vi "CRYReport Part TX LIB.vi"(6 "Control Ref":refnum<k7>, 7 "sAction":string, 8 "nData":i32, 9 "sData":string, 10 "TXTextControl":refnum<k7>, 11 "cFrame":T1) -> (0 "nData_Out":i32, 1 "sData_Out":string, 3 "cFrame_Out":T1)   [LabVIEW 2013]
uses:
  CRYReport Global.vi
  CRYWindow/SubVI/CRYMain Sub Window Global.vi
  PrintTxDocDLL.dll
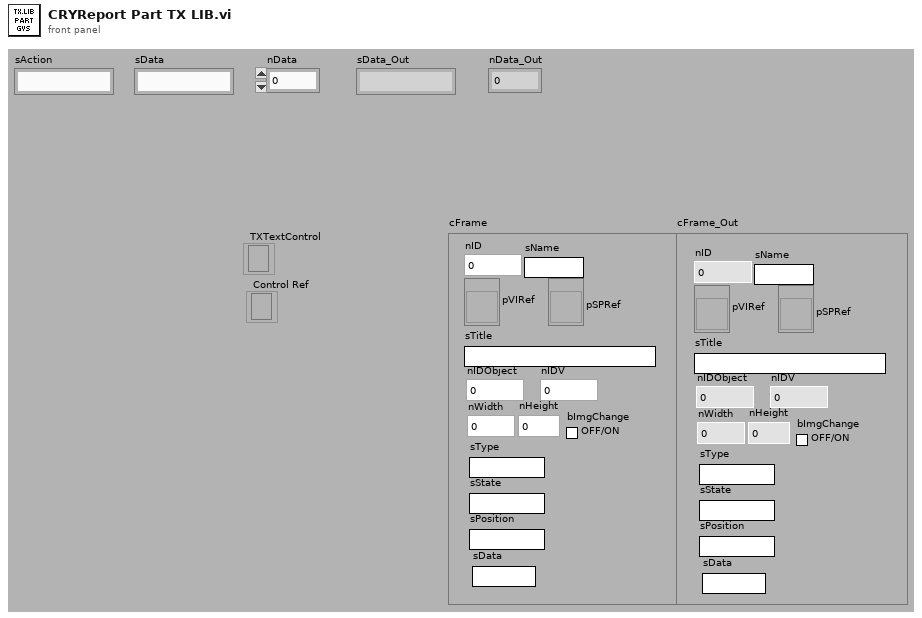
[diagram p1: front panel]
types:
  T1 = cluster{"nID":i16, "sName":string, "pVIRef":refnum<vi>, "pSPRef":refnum<vi>, "sTitle":string, "nIDObject":i16, "nIDV":i16, "nWidth":i16, "nHeight":i16, "bImgChange":bool, "sType":string, "sState":string, "sPosition":string, "sData":string}
  T2 = typedef "LVRectTypeDef.ctl" = cluster{"Left":i16, "Top":i16, "Right":i16, "Bottom":i16}
  T3 = cluster{"nType":i32, "nParent":i32, "pVIW":refnum<vi>, "pSPW":refnum<vi>, "nTypeF":i32, "pVIF":refnum<vi>, "pSPF":refnum<vi>, "nIDSpliter":i32, "nProperty":i32, "Bound":T2, "nID":i32, "nData":i32, "sData":string, "pWVI":refnum<vi>, "sTitle":string, "cPages":cluster{"nPage":i32, "sTitle":string, "sIcon":string, "pVI":refnum<vi>, "nID":i32}[], "pTab":refnum<vi>, "nIDPages":i32[], "pSPT":refnum<vi>, "sTemp":string, "nDockID":i32, "nDockLR":i32, "sIcon":string}
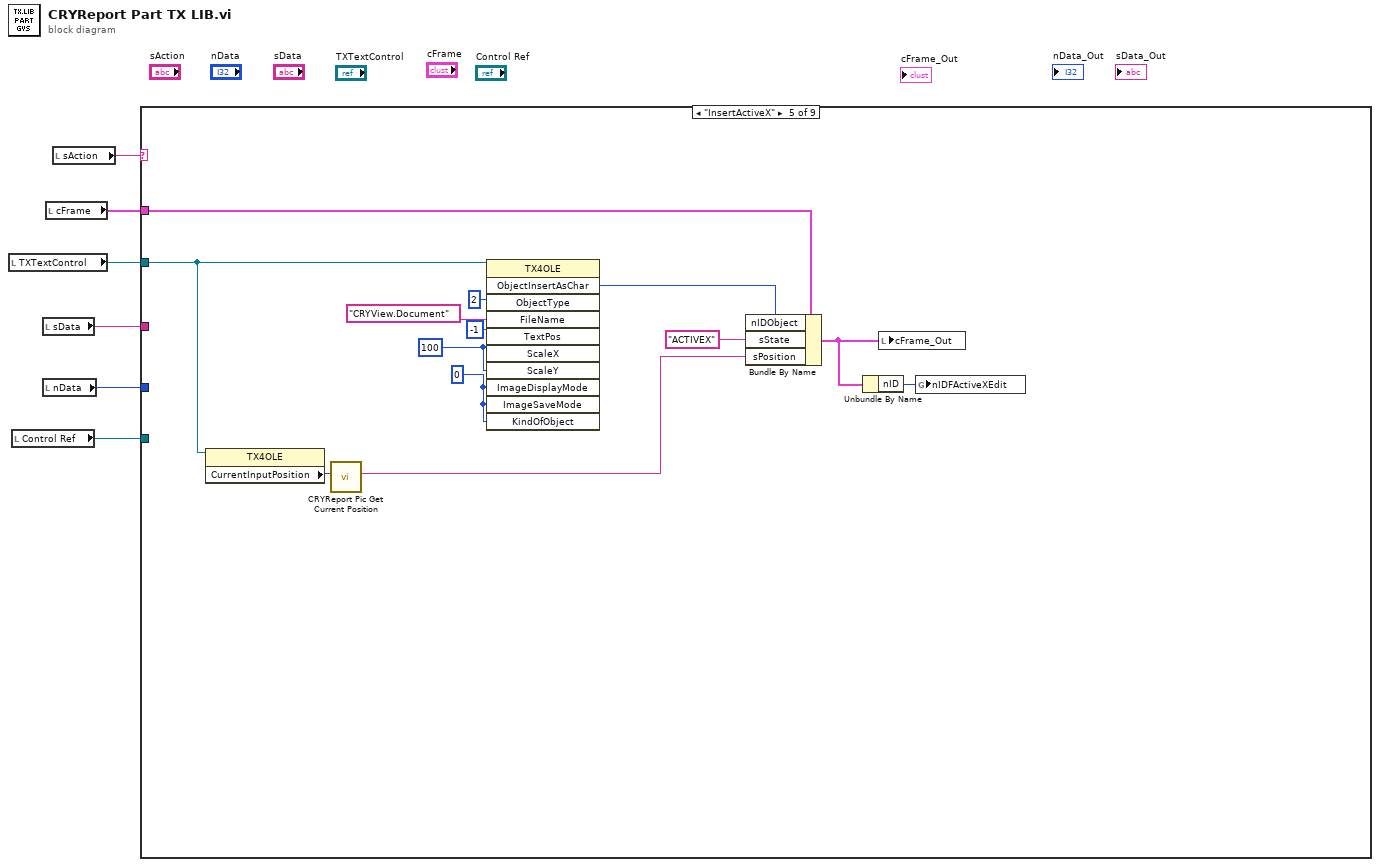
[diagram p0: block diagram]
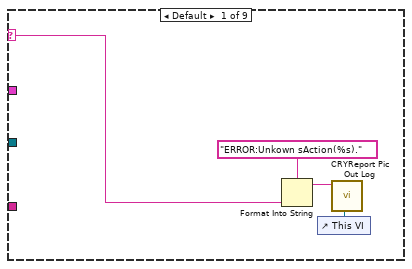
[diagram p2: hidden frame]
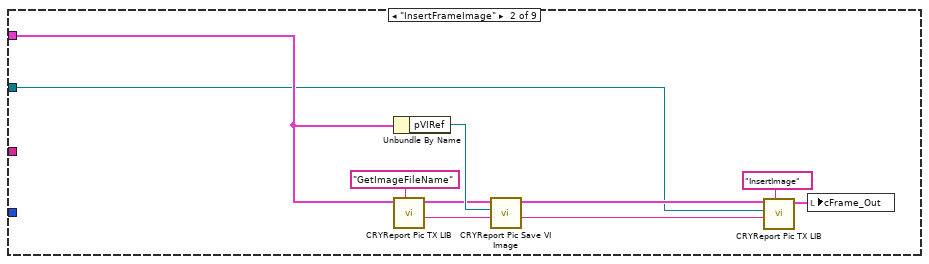
[diagram p3: hidden frame]
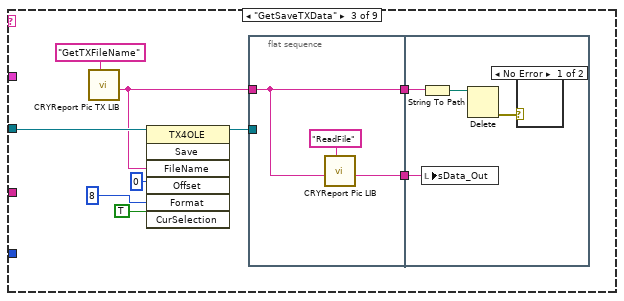
[diagram p4: hidden frame]
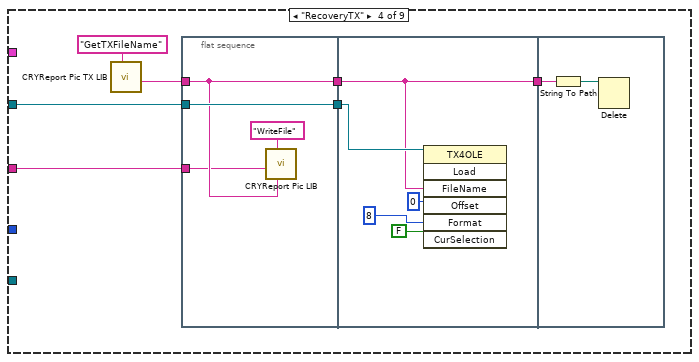
[diagram p6: hidden frame]
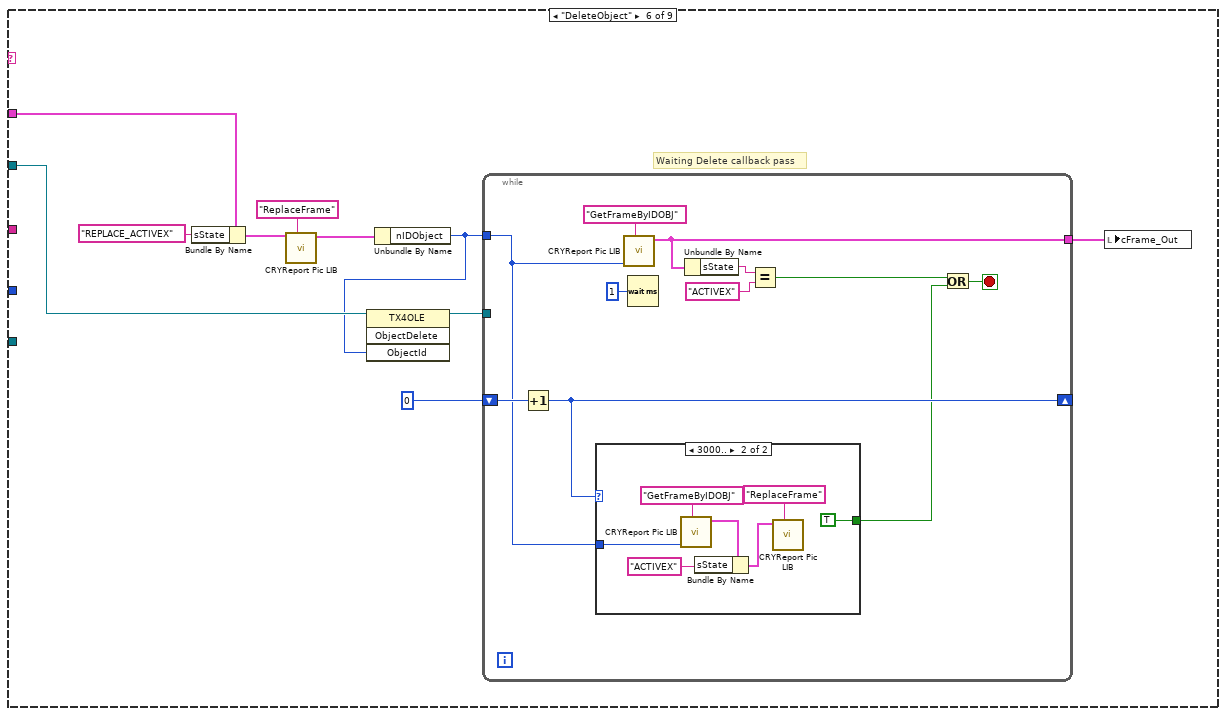
[diagram p7: hidden frame]
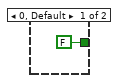
[diagram p8: hidden frame]
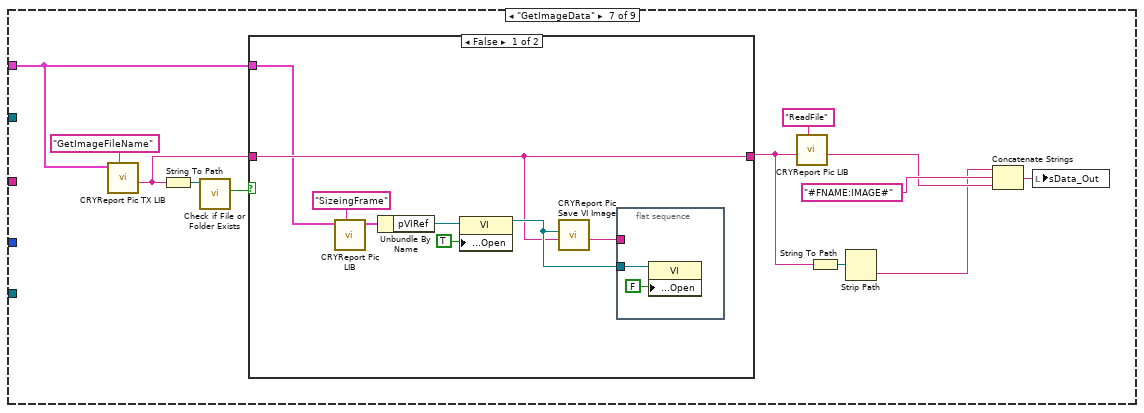
[diagram p9: hidden frame]
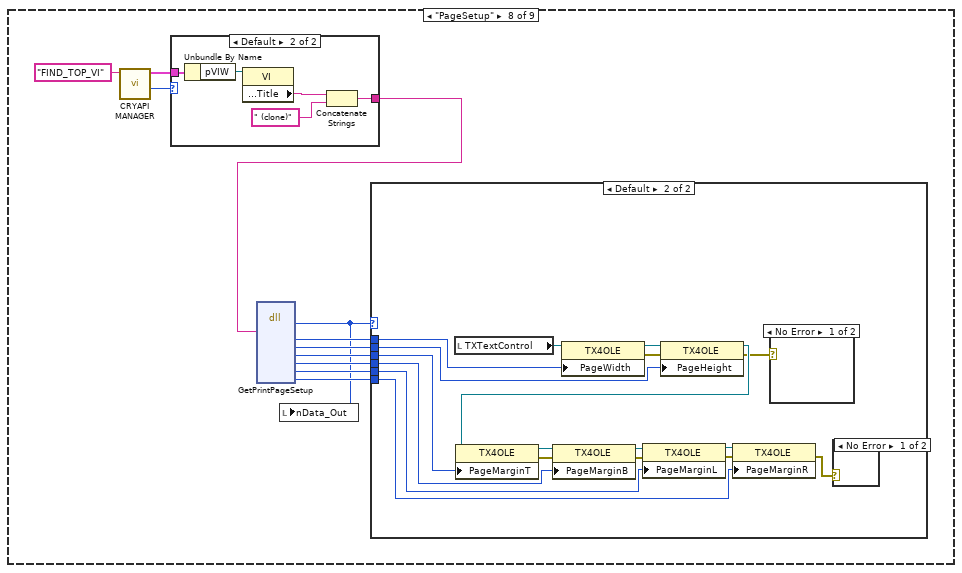
[diagram p11: hidden frame]
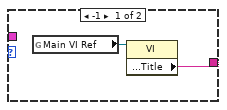
[diagram p15: hidden frame]
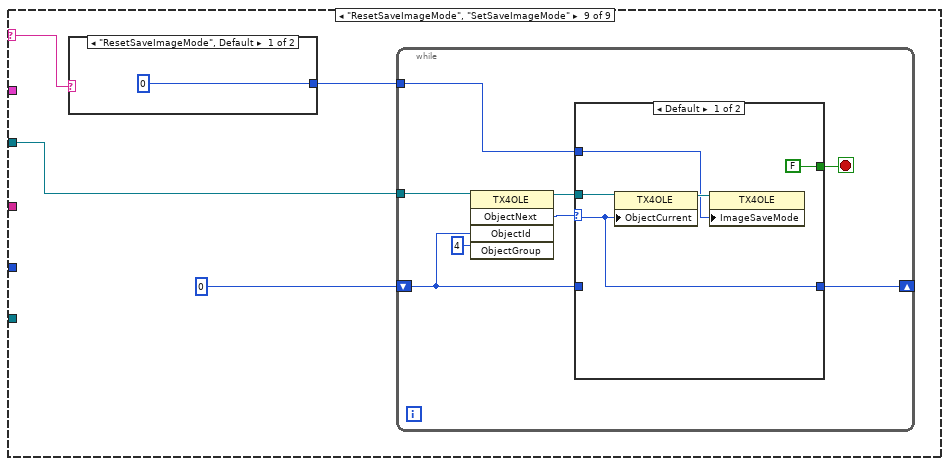
[diagram p16: hidden frame]
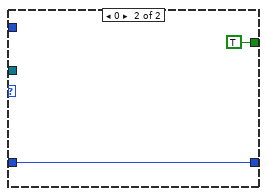
[diagram p17: hidden frame]
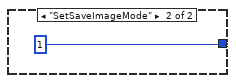
[diagram p18: hidden frame]
diagram:
  n1 = local read "TXTextControl"() -> (w2:refnum<k7>)
  n2 = local read "Control Ref"() -> (w1:refnum<k7>)
  n3 = local read "sData"() -> (w5:string)
  n4 = local read "nData"() -> (w4:i32)
  n5 = local read "cFrame"() -> (w3:T1)
  n6 = local read "sAction"() -> (w6:string)
  n7 = case shown="\"InsertActiveX\"" w6 {
    selector: w6 -> [w8 _ _ _ _ _ _ _ w159]
    tunnel: w5 -> [_ _ _ w41 _ _ _ _ _]
    tunnel: w4 -> [_ _ _ _ _ _ _ _ _]
    tunnel: w3 -> [_ w20 _ _ w56 w73 w105 _ _]
    tunnel: w2 -> [_ w15 w27 w40 w55 w74 _ _ w158]
    tunnel: w1 -> [_ _ _ _ _ _ _ _ _]
    frame Default {
      n8 = Format Into String(format string="ERROR:Unkown sAction(%s).", w8) -> (resulting string=w7:string)  [unwired: 2 in, 1 out]
      n9 = control-ref of="This VI"() -> (w10:refnum<vi>)
      n10 = call "CRYReport Pic Out Log.vi"("vi reference"=w10, "sData"=w7) -> ()  [unwired: 10 in]
    }
    frame "InsertFrameImage" {
      n11 = Unbundle By Name(w20) -> ("pVIRef"=w14:refnum<vi>)
      n12 = call "CRYReport Pic TX LIB.vi"("sAction"="GetImageFileName", "cFrame"=w20) -> ("sData_Out"=w12:string, "cFrame_Out"=w11:T1)  [unwired: 7 in, 1 out]
      n13 = call "CRYReport Pic Save VI Image.vi"("sData"=w12, "pVIRef"=w14, "cFrame"=w11) -> ("sData_Out"=w19:string, "cFrame_Out"=w18:T1)  [unwired: 7 in]
      n14 = call "CRYReport Pic TX LIB.vi"("sAction"="InsertImage", "sData"=w19, "TXTextControl"=w15, "cFrame"=w18) -> ("cFrame_Out"=w16:T1)  [unwired: 5 in, 2 out]
      n15 = local write "cFrame_Out"(w16) -> ()
    }
    frame "GetSaveTXData" {
      n16 = call "CRYReport Pic TX LIB.vi"("sAction"="GetTXFileName") -> ("sData_Out"=w24:string)  [unwired: 8 in, 2 out]
      n17 = invoke class="TX4OLE" method="Save"(reference=w27, "FileName"=w24, "Offset"=0, "Format"=8 ("nData"), "CurSelection"=TRUE) -> (reference out=w23:refnum<k7>)  [unwired: 2 in, 6 out]
      n18 = flat-sequence {
        tunnel: w24 -> [w31]
        tunnel: w23 -> [_]
        tunnel: [w31] -> w22
        tunnel: [w30] -> w21
        tunnel: w22 -> [w36]
        tunnel: w21 -> [w34]
        frame #0 {
          n19 = call "CRYReport Pic LIB.vi"("sAction"="ReadFile", "sData"=w31) -> ("sData_Out"=w30:string)  [unwired: 6 in, 3 out]
        }
        frame #1 {
          n20 = String To Path(string=w36) -> (path=w35:path)
          n21 = local write "sData_Out"(w34) -> ()
          n22 = Delete(path (use dialog)=w35) -> (error out=w33:errorcluster)  [unwired: 4 in, 2 out]
          n23 = case shown="No Error" w33 {
            frame No Error {
            }
            frame Error {
            }
          }
        }
      }
    }
    frame "RecoveryTX" {
      n24 = call "CRYReport Pic TX LIB.vi"("sAction"="GetTXFileName") -> ("sData_Out"=w42:string)  [unwired: 8 in, 2 out]
      n25 = flat-sequence {
        tunnel: w41 -> [w44]
        tunnel: w42 -> [w45]
        tunnel: w40 -> [w47]
        tunnel: [w45] -> w39
        tunnel: [w47] -> w38
        tunnel: w39 -> [w48]
        tunnel: w38 -> [w49]
        tunnel: [w48] -> w37
        tunnel: w37 -> [w53]
        frame #0 {
          n26 = call "CRYReport Pic LIB.vi"("sOption"=w45, "sAction"="WriteFile", "sData"=w44) -> ()  [unwired: 5 in, 4 out]
        }
        frame #1 {
          n27 = invoke class="TX4OLE" method="Load"(reference=w49, "FileName"=w48, "Offset"=0, "Format"=8 ("nData"), "CurSelection"=FALSE) -> ()  [unwired: 2 in, 7 out]
        }
        frame #2 {
          n28 = String To Path(string=w53) -> (path=w54:path)
          n29 = Delete(path (use dialog)=w54) -> ()  [unwired: 4 in, 3 out]
        }
      }
    }
    frame "InsertActiveX" {
      w62 = i16 0 ("ImageDisplayMode")
      w63 = i16 100 ("ScaleX")
      n30 = property class="TX4OLE"(reference=w55) -> ("CurrentInputPosition"=w57:variant)  [unwired: 1 in, 2 out]
      n31 = call "CRYReport Pic Get Current Position.vi"("CurrentInputPosition"=w57) -> ("sData_Out"=w61:string)  [unwired: 9 in, 1 out]
      n32 = invoke class="TX4OLE" method="ObjectInsertAsChar"(reference=w55, "ObjectType"=2, "FileName"="CRYView.Document", "TextPos"=-1, "ScaleX"=w63, "ScaleY"=w63, "ImageDisplayMode"=w62, "ImageSaveMode"=w62, "KindOfObject"=w62) -> ("ObjectInsertAsChar"=w67:i16)  [unwired: 2 in, 10 out]
      n33 = Bundle By Name(cluster=w56, "nIDObject"=w67, "sState"="ACTIVEX", "sPosition"=w61) -> (w59:T1)
      n34 = Unbundle By Name(w59) -> ("nID"=w58:i16)
      n35 = local write "cFrame_Out"(w59) -> ()
      n36 = global write "CRYReport Global.vi" "nIDFActiveXEdit"(w58) -> ()
    }
    frame "DeleteObject" {
      # "Waiting Delete callback pass"
      n37 = Bundle By Name(cluster=w73, "sState"="REPLACE_ACTIVEX") -> (w76:T1)
      n38 = call "CRYReport Pic LIB.vi"("sAction"="ReplaceFrame", "cFrame"=w76) -> ("cFrame_Out"=w72:T1)  [unwired: 6 in, 3 out]
      n39 = Unbundle By Name(w72) -> ("nIDObject"=w70:i16)
      n40 = invoke class="TX4OLE" method="ObjectDelete"(reference=w74, "ObjectId"=w70) -> (reference out=w71:refnum<k7>)  [unwired: 2 in, 3 out]
      n41 = while {
        tunnel: w71 -> [_]
        tunnel: w70 -> [w81]
        tunnel: [w84] -> w69
        shift-right: [w82] -> _
        shift-left: 0 -> [w83]
        stop <- w80 stop-if-true
        n42 = Increment(x=w83) -> (x+1=w82:i32)
        n43 = case shown="3000.." w82 {
          tunnel: w81 -> [_ w95]
          tunnel: [FALSE TRUE] -> w78
          frame 0, Default {
          }
          frame 3000.. {
            n44 = call "CRYReport Pic LIB.vi"("sAction"="GetFrameByIDOBJ", "nData"=w95) -> ("cFrame_Out"=w94:T1)  [unwired: 6 in, 3 out]
            n45 = Bundle By Name(cluster=w94, "sState"="ACTIVEX") -> (w91:T1)
            n46 = call "CRYReport Pic LIB.vi"("sAction"="ReplaceFrame", "cFrame"=w91) -> ()  [unwired: 6 in, 4 out]
          }
        }
        n47 = call "CRYReport Pic LIB.vi"("sAction"="GetFrameByIDOBJ", "nData"=w81) -> ("cFrame_Out"=w84:T1)  [unwired: 6 in, 3 out]
        n48 = Wait (ms)(milliseconds to wait=u32 1) -> ()  [unwired: 1 out]
        n49 = Unbundle By Name(w84) -> ("sState"=w88:string)
        n50 = Equal?(x=w88, y="ACTIVEX" ("sState")) -> (x = y?=w79:bool)
        n51 = Or(x=w79, y=w78) -> (x .or. y?=w80:bool)
      }
      n52 = local write "cFrame_Out"(w69) -> ()
    }
    frame "GetImageData" {
      n53 = call "CRYReport Pic TX LIB.vi"("sAction"="GetImageFileName", "cFrame"=w105) -> ("sData_Out"=w104:string)  [unwired: 7 in, 2 out]
      n54 = String To Path(string=w104) -> (path=w108:path)
      n55 = call <vilib>:"Check if File or Folder Exists.vi"("path"=w108) -> ("file or folder exists?"=w107:bool)  [unwired: 8 in, 2 out]
      n56 = case shown="False" w107 {
        tunnel: w105 -> [w111 _]
        tunnel: w104 -> [w113 w119]
        tunnel: [w113 w119] -> w98
        frame False {
          n57 = call "CRYReport Pic LIB.vi"("sAction"="SizeingFrame", "cFrame"=w111) -> ("cFrame_Out"=w110:T1)  [unwired: 6 in, 3 out]
          n58 = Unbundle By Name(w110) -> ("pVIRef"=w109:refnum<vi>)
          n59 = property class="VI"(reference=w109, "Front Panel.Open"=TRUE ("Front Panel Window:Open")) -> (reference out=w115:refnum<vi>)  [unwired: 1 in, 1 out]
          n60 = call "CRYReport Pic Save VI Image.vi"("sData"=w113, "pVIRef"=w115) -> ("sData_Out"=w114:string)  [unwired: 8 in, 1 out]
          n61 = flat-sequence {
            tunnel: w115 -> [w117]
            tunnel: w114 -> [_]
            frame #0 {
              n62 = property class="VI"(reference=w117, "Front Panel.Open"=FALSE ("Front Panel Window:Open")) -> ()  [unwired: 1 in, 2 out]
            }
          }
        }
        frame True {
        }
      }
      n63 = call "CRYReport Pic LIB.vi"("sAction"="ReadFile", "sData"=w98) -> ("sData_Out"=w101:string)  [unwired: 6 in, 3 out]
      n64 = String To Path(string=w98) -> (path=w99:path)
      n65 = Strip Path(path=w99) -> (name=w97:string)  [unwired: 1 out]
      n66 = Concatenate Strings(w97, "#FNAME:IMAGE#" ("regular expression"), w101) -> (w100:string)
      n67 = local write "sData_Out"(w100) -> ()
    }
    frame "PageSetup" {
      n68 = call "CRYAPI MANAGER.vi"("sAction"="FIND_TOP_VI") -> ("nData_Out"=w129:i32, "tFrame_Out"=w128:T3)  [unwired: 9 in]
      n69 = case shown="Default" w129 {
        tunnel: w128 -> [_ w155]
        tunnel: [w149 w151] -> w120
        frame -1 {
          n70 = global read "CRYMain Sub Window Global.vi" "Main VI Ref"() -> (w150:refnum<vi>)
          n71 = property class="VI"(reference=w150) -> ("Front Panel.Title"=w149:string)  [unwired: 1 in, 2 out]
        }
        frame Default {
          n72 = Unbundle By Name(w155) -> ("pVIW"=w154:refnum<vi>)
          n73 = property class="VI"(reference=w154) -> ("Front Panel.Title"=w153:string)  [unwired: 1 in, 2 out]
          n74 = Concatenate Strings(w153, " (clone)" ("string")) -> (w151:string)
        }
      }
      n75 = dll-call lib="D:/LabView_Project/CRY6181/CRYDocument/PrintTxDocDLL.dll" fn="GetPrintPageSetup"("szTitle"=w120) -> ("return type"=w121:i32, "nW"=w127:i32, "nH"=w126:i32, "nT"=w125:i32, "nB"=w124:i32, "nL"=w123:i32, "nR"=w122:i32)  [unwired: 3 in, 9 out]
      n76 = local write "nData_Out"(w121) -> ()
      n77 = case shown="Default" w121 {
        tunnel: w127 -> [_ w138]
        tunnel: w126 -> [_ w137]
        tunnel: w125 -> [_ w136]
        tunnel: w124 -> [_ w135]
        tunnel: w123 -> [_ w134]
        tunnel: w122 -> [_ w133]
        frame 0 {
        }
        frame Default {
          n78 = local read "TXTextControl"() -> (w148:refnum<k7>)
          n79 = property class="TX4OLE"(reference=w148, "PageWidth"=w138) -> (reference out=w147:refnum<k7>, error out=w146:errorcluster)  [unwired: 1 in]
          n80 = property class="TX4OLE"(reference=w147, error in=w146, "PageHeight"=w137) -> (reference out=w139:refnum<k7>, error out=w131:errorcluster)
          n81 = property class="TX4OLE"(reference=w139, "PageMarginT"=w136) -> (reference out=w145:refnum<k7>, error out=w144:errorcluster)  [unwired: 1 in]
          n82 = property class="TX4OLE"(reference=w145, error in=w144, "PageMarginB"=w135) -> (reference out=w143:refnum<k7>, error out=w142:errorcluster)
          n83 = property class="TX4OLE"(reference=w143, error in=w142, "PageMarginL"=w134) -> (reference out=w141:refnum<k7>, error out=w140:errorcluster)
          n84 = property class="TX4OLE"(reference=w141, error in=w140, "PageMarginR"=w133) -> (error out=w132:errorcluster)  [unwired: 1 out]
          n85 = case shown="No Error" w131 {
            frame No Error {
            }
            frame Error {
            }
          }
          n86 = case shown="No Error" w132 {
            frame No Error {
            }
            frame Error {
            }
          }
        }
      }
    }
    frame "ResetSaveImageMode", "SetSaveImageMode" {
      n87 = case shown="\"ResetSaveImageMode\", Default" w159 {
        tunnel: [0 1] -> w156
        frame "ResetSaveImageMode", Default {
        }
        frame "SetSaveImageMode" {
        }
      }
      n88 = while {
        tunnel: w158 -> [w167]
        tunnel: w156 -> [w164]
        shift-right: [w161] -> _
        shift-left: 0 -> [w162]
        stop <- w163 stop-if-true
        n89 = invoke class="TX4OLE" method="ObjectNext"(reference=w167, "ObjectId"=w162, "ObjectGroup"=i16 4) -> (reference out=w165:refnum<k7>, "ObjectNext"=w160:i16)  [unwired: 2 in, 3 out]
        n90 = case shown="Default" w160 {
          selector: w160 -> [w168 _]
          tunnel: w165 -> [w172 _]
          tunnel: w164 -> [w170 _]
          tunnel: [FALSE TRUE] -> w163
          tunnel: w162 -> [_ w173]
          tunnel: [w168 w173] -> w161
          frame Default {
            n91 = property class="TX4OLE"(reference=w172, "ObjectCurrent"=w168) -> (reference out=w171:refnum<k7>)  [unwired: 1 in, 1 out]
            n92 = property class="TX4OLE"(reference=w171, "ImageSaveMode"=w170) -> ()  [unwired: 1 in, 2 out]
          }
          frame 0 {
          }
        }
      }
    }
  }
